vi "sub_Find_Sync_Index.vi"(7 "samples per symbol (16)":i32=16, 8 "error in (no error)":errorcluster, 9 "matched filter coefficients":dbl[](array[numeric]) format="%^.2e", 10 "Sync Sequence Waveform":cdb[](array[numeric]), 11 "Input Complex Waveform":T1={"t0"=0.0, "dt"=1.0, "Y"=[]} {"Y" format="%.3f"; "dt" format="%^.2e"; "t0" format="%.4f"}) -> (0 "error out":errorcluster, 2 "Max Xcorr Abs Value":dbl, 3 "Max Xcorr Index":i32)   [LabVIEW 2014]
uses:
  <vilib>/addons/Modulation/Analog/controls/Complex Data Waveform.ctl
  <vilib>/Analysis/2dsp.llb/1D Cross Correlation (CDB).vi
  <vilib>/addons/Modulation/Digital/General/MT Apply Matched Filter (Generic).vi
  <vilib>/Analysis/NI_AALPro.lvlib
  <vilib>/addons/Modulation/niDMT.lvlib
  <vilib>/addons/Modulation/niAMT.lvlib
panel:
  out "Max Xcorr Complex":cdb
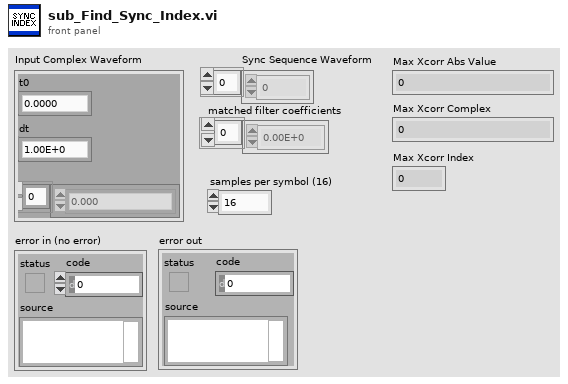
[diagram p1: front panel]
types:
  T1 = typedef "niAMT.lvlib/Complex Data Waveform.ctl" = cluster{"t0":dbl, "dt":dbl, "Y":cdb[]}
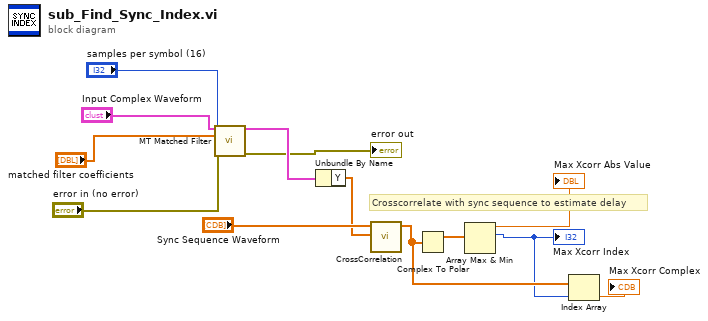
[diagram p0: block diagram]
diagram:
  # "Crosscorrelate with sync sequence to estimate delay"
  n1 = call-poly <vilib>:"MT Matched Filter.vi"("input complex waveform"="Input Complex Waveform", "matched filter coefficients"="matched filter coefficients", "samples per symbol (16)"="samples per symbol (16)", "error in (no error)"="error in (no error)") -> ("output complex waveform"=w10:T1, "error out"=→"error out":errorcluster)  [unwired: 10 in]
  n2 = Unbundle By Name(w10) -> ("Y"=w12:cdb[])
  n3 = call-poly <vilib>:"CrossCorrelation.vi"("Y"=w12, "X"="Sync Sequence Waveform") -> ("Rxy"=w3:cdb[])  [unwired: 8 in, 1 out]
  n4 = Complex To Polar(r * e^(i*theta)=w3) -> (r=w4:dbl[])  [unwired: 1 out]
  n5 = Array Max & Min(array=w4) -> (max value=→"Max Xcorr Abs Value":dbl, max index (indices)=w2:i32)  [unwired: 2 out]
  "Max Xcorr Index" <- w2
  n6 = Index Array(array=w3, index=w2) -> (element=→"Max Xcorr Complex":cdb)
